vi "Actor Core.vi"(8 "error in":errorcluster, 11 "WT1600 in":refnum<class "WT1600.lvclass">) -> (0 "error out":errorcluster, 3 "Actor out":refnum<class "Actor.lvclass">)   [LabVIEW 2013, in "WT1600.lvlib" / "WT1600.lvclass"]
doc: "(<B>Filename</B>: Actor Framework.lvlib:Actor.lvclass:Actor Core.vi)\n\nReceives messages to the actor, reacts to them, and initiates any error handling that may shut the actor down.\n\nDescendant classes may override this VI to append parallel tasks for the actor to complete while it handles messages. Overrides use the Call Parent Method node."
uses:
  WT1600.lvclass
  <vilib>/ActorFramework/Actor/Actor.lvclass
  1600Card/1600Card/1600 Card Actor.lvclass
  WT1600.lvclass/WT1600.ctl
  <vilib>/ActorFramework/Actor/Actor.lvclass/Actor.ctl
  <vilib>/ActorFramework/Message Enqueuer/Message Enqueuer.lvclass/Message Enqueuer.ctl
  Observer Pattern Actor Template/Subject/Subject.lvclass
  1600Card/1600Card/1600 Card Actor.lvclass/1600 Card Actor.ctl
  Observer Pattern Actor Template/Subject Messages/Register Observer Msg/Register Observer Msg.lvclass/Register Observer Msg.ctl
  <vilib>/ActorFramework/Message Enqueuer/Init from Existing Queue.vi
  <vilib>/ActorFramework/Message Enqueuer/Enqueue.vi
  <vilib>/ActorFramework/Message Priority Queue/Priority Enqueue.vi
  <vilib>/ActorFramework/Message Enqueuer/Message Enqueuer.lvclass
  WT1600 Messages/Measure Msg/Measure Msg.lvclass
  Observer Pattern Actor Template/Subject Messages/Register Observer Msg/Register Observer Msg.lvclass
  WT1600.lvlib
panel:
  out "W-Hr":dbl
  out "Freq.":dbl
  out "Power":dbl
  out "Current":dbl
  out "Voltage":dbl
  in  "Card Number":u8=1 max=1
  in  "Array":dbl[](array[numeric])
  in  "Card Cluster":T1
  in  "New Card":bool
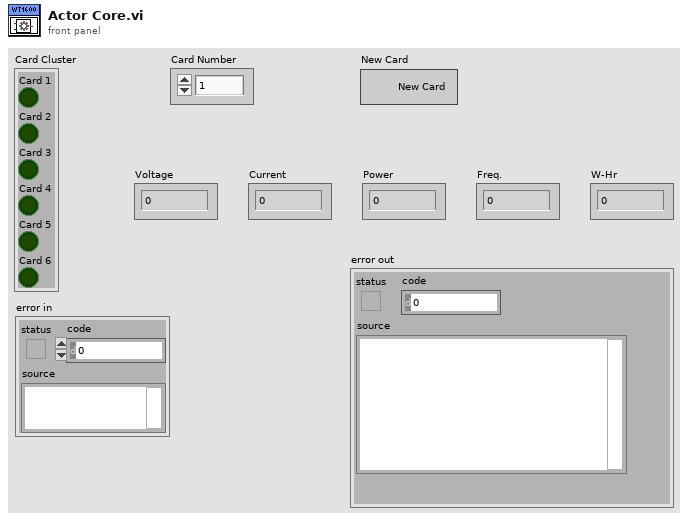
[diagram p1: front panel]
types:
  T1 = cluster{"Card 1":bool, "Card 2":bool, "Card 3":bool, "Card 4":bool, "Card 5":bool, "Card 6":bool}
  T2 = cluster{"Card Cluster[0]":bool, "Card Cluster[1]":bool, "Card Cluster[2]":bool, "Card Cluster[3]":bool, "Card Cluster[4]":bool, "Card Cluster[5]":bool}
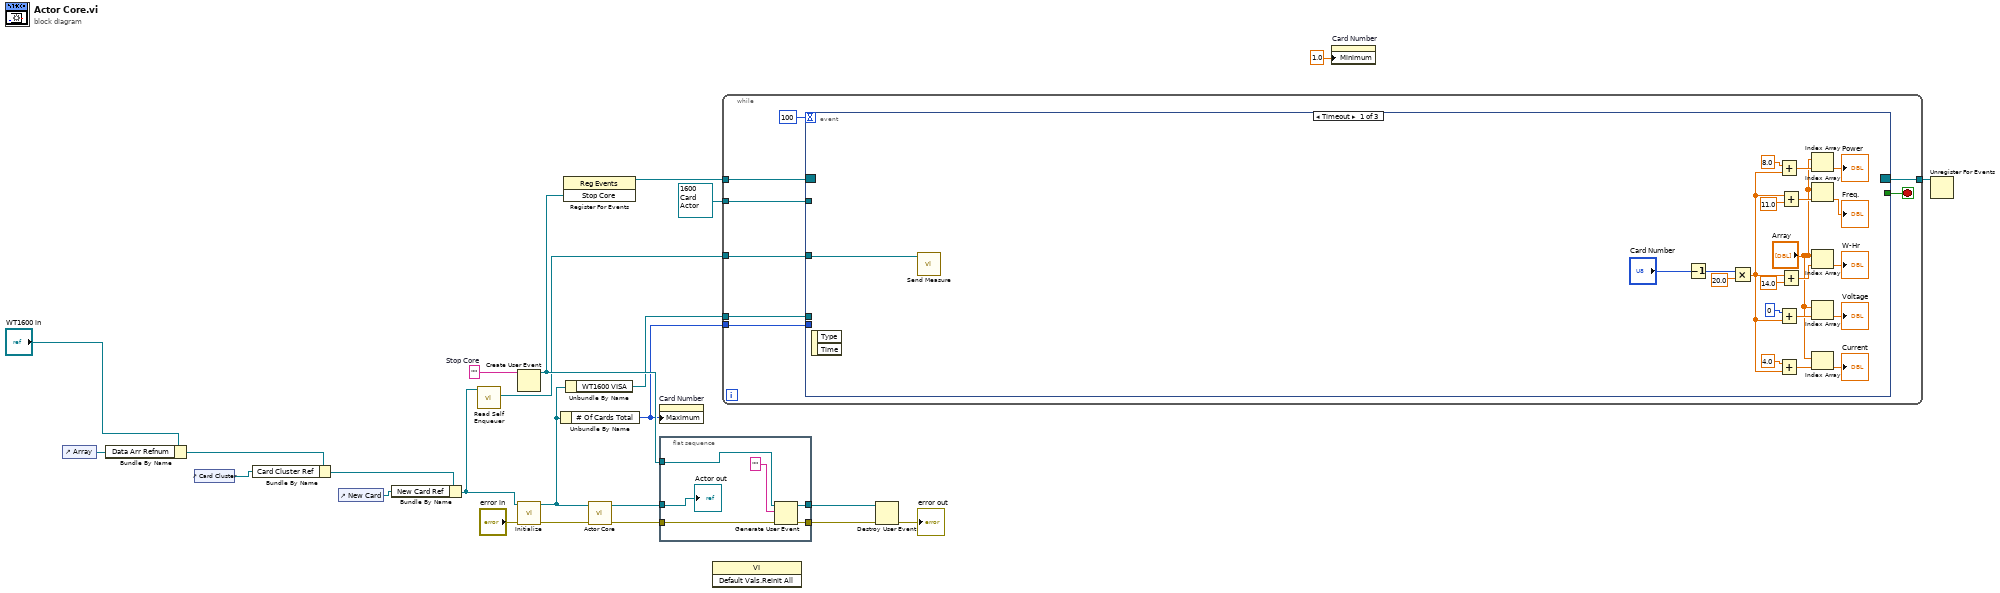
[diagram p0: block diagram]
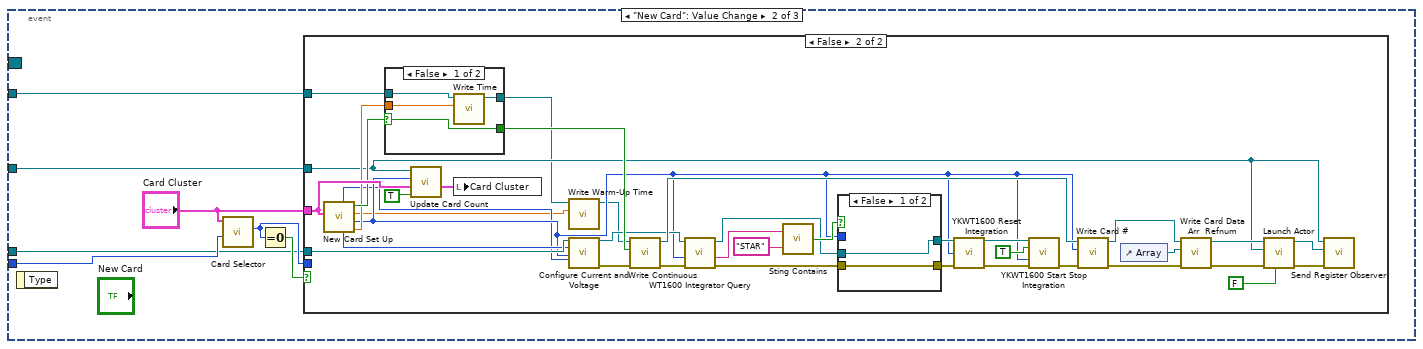
[diagram p2: hidden frame]
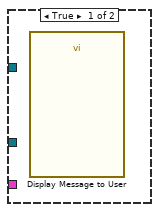
[diagram p3: hidden frame]
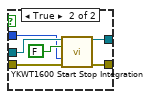
[diagram p5: hidden frame]
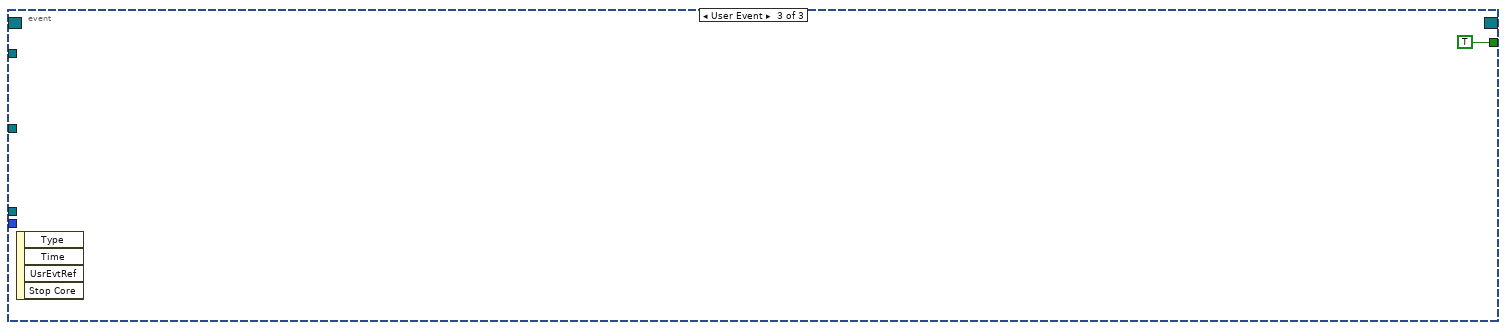
[diagram p6: hidden frame]
diagram:
  w17 = ""  # Stop Core
  n1 = control-ref of="Array"() -> (w5:refnum<vi>)
  n2 = Bundle By Name(cluster="WT1600 in", "Data Arr Refnum"=w5) -> (w6:refnum<class "WT1600.lvclass">)
  n3 = control-ref of="Card Cluster"() -> (w9:refnum<vi>)
  n4 = Bundle By Name(cluster=w6, "Card Cluster Ref"=w9) -> (w10:refnum<class "WT1600.lvclass">)
  n5 = control-ref of="New Card"() -> (w11:refnum<vi>)
  n6 = Bundle By Name(cluster=w10, "New Card Ref"=w11) -> (w8:refnum<class "WT1600.lvclass">)
  n7 = call <vilib>:"Read Self Enqueuer.vi"("Actor"=w8) -> ("Self Enqueuer"=w13:refnum<class "Message Enqueuer.lvclass">)  [unwired: 10 in]
  n8 = Create User Event(user event datatype=w17) -> (user event=w15:refnum<user-event>)  [unwired: 1 in, 1 out]
  n9 = call-dynamic "Initialize.vi"("WT1600.lvlib:WT1600.lvclass"=w8, "error in (no error)"="error in") -> ("WT1600.lvlib:WT1600.lvclass"=w3:refnum<class "WT1600.lvclass">, "error out (no error)"=w23:errorcluster)  [unwired: 11 in, 1 out]
  n10 = Unbundle By Name(w3) -> ("# Of Cards Total"=w1:i32)
  n11 = register-events(w15) -> (reference out=w16:refnum<event-registration>)  [unwired: 2 in, 1 out]
  n12 = Unbundle By Name(w3) -> ("WT1600 VISA"=w2:refnum<visa-resource-name>)
  n13 = call-parent "Actor Core.vi"("error in"=w23, "Actor in"=w3) -> ("error out"=w22:errorcluster, "Actor out"=w21:refnum<class "Actor.lvclass">)  [unwired: 8 in]
  n14 = property on="Card Number" class="DigNum (strict)"("Maximum"=w1) -> ()  [unwired: 2 in, 2 out]
  n15 = flat-sequence {
    tunnel: w22 -> [w27]
    tunnel: w21 -> [w30]
    tunnel: [w29] -> w20
    tunnel: [w28] -> w19
    tunnel: w15 -> [w26]
    frame #0 {
      n16 = Generate User Event(user event=w26, event data cluster="" ("event data"), error in=w27) -> (user event out=w29:refnum<user-event>, error out=w28:errorcluster)  [unwired: 1 in]
      "Actor out" <- w30
    }
  }
  n17 = invoke class="VI" method="Default Vals.Reinit All"() -> ()  [unwired: 3 in, 3 out]
  n18 = while {
    tunnel: w16 -> [w38]
    tunnel: [w37] -> w14
    tunnel: w13 -> [w33]
    tunnel: refnum<class "1600 Card Actor.lvclass"> refnum ("WT1600.lvlib:1600Card.lvlib:1600 Card Actor.lvclass") -> [w34]
    tunnel: w1 -> [w32]
    tunnel: w2 -> [w31]
    stop <- w36 stop-if-true
    n19 = event shown="[0] Timeout" {
      selector: w38 -> [_ _ _]
      dyn-events: [_ _ _] -> w37
      timeout: 100 -> [_ _ _]
      tunnel: [_ _ TRUE] -> w36
      tunnel: w34 -> [_ w66 _]
      tunnel: w33 -> [w59 w65 _]
      tunnel: w32 -> [_ w63 _]
      tunnel: w31 -> [_ w60 _]
      event Timeout {
        n20 = event-data() -> ()  [unwired: 1 in, 2 out]
        n21 = call "Send Measure.vi"("Message Enqueuer"=w59) -> ()  [unwired: 9 in, 2 out]
        n22 = Decrement(x="Card Number") -> (x-1=w58:u8)
        n23 = Multiply(x=w58, y=20.0) -> (x*y=w49:dbl)
        n24 = Add(x=8.0, y=w49) -> (x+y=w51:dbl)
        n25 = Add(x=0 ("index"), y=w49) -> (x+y=w54:dbl)
        n26 = Add(x=4.0, y=w49) -> (x+y=w53:dbl)
        n27 = Add(x=w49, y=11.0) -> (x+y=w47:dbl)
        n28 = Add(x=w49, y=14.0) -> (x+y=w46:dbl)
        n29 = Index Array(array="Array", index=w51) -> (element=→"Power":dbl)
        n30 = Index Array(array="Array", index=w47) -> (element=→"Freq.":dbl)
        n31 = Index Array(array="Array", index=w46) -> (element=→"W-Hr":dbl)
        n32 = Index Array(array="Array", index=w54) -> (element=→"Voltage":dbl)
        n33 = Index Array(array="Array", index=w53) -> (element=→"Current":dbl)
      }
      event "New Card": Value Change {
        n34 = event-data() -> ()  [unwired: 1 in, 1 out]
        n35 = call "Card Selector.vi"("# Of Cards Total"=w63, "Card Cluster"="Card Cluster") -> ("Card to use"=w62:i32)  [unwired: 9 in]
        n36 = Equal To 0?(x=w62) -> (x = 0?=w64:bool)
        n37 = case shown="False" w64 {
          tunnel: w66 -> [_ w77]
          tunnel: w65 -> [_ w76]
          tunnel: w62 -> [_ _]
          tunnel: "Card Cluster" -> [_ w97]
          tunnel: w60 -> [_ w75]
          frame True {
            n38 = call "Display Message to User"() -> ()  [unwired: 10 in, 2 out]
          }
          frame False {
            n39 = call "New Card Set Up.vi"("Card Cluster"=w97) -> ("Measurement Time 2"=w78:dbl, "Card chosen"=w71:i32, "Warm Up Time 2"=w67:dbl, "Continuous?"=w80:bool, "V Range (12: 1000) 2"=w72:u16, "A Range (9: 5A) 2"=w70:u16)  [unwired: 5 in]
            n40 = case shown="False" w80 {
              selector: w80 -> [w108 w110]
              tunnel: [w108 w110] -> w79
              tunnel: w78 -> [w107 _]
              tunnel: w77 -> [w106 w109]
              tunnel: [w105 w109] -> w69
              frame False {
                n41 = call "Write Time .vi"("Time"=w107, "1600 Card Actor in"=w106) -> ("1600 Card Actor out"=w105:refnum<class "1600 Card Actor.lvclass">)  [unwired: 8 in, 1 out]
              }
              frame True {
              }
            }
            n42 = call "Update Card Count.vi"("new element/subarray"=TRUE ("Open Actor Core front panel? (F)"), "cluster in"=w97, "# in"=w71, "Message Enqueuer"=w76) -> ("cluster out"=w102:T2)  [unwired: 7 in]
            n43 = local write "Card Cluster"(w102) -> ()
            n44 = call "Write Warm-Up Time.vi"("Warm-Up Time"=w67, "1600 Card Actor in"=w69) -> ("1600 Card Actor out"=w68:refnum<class "1600 Card Actor.lvclass">)  [unwired: 8 in, 1 out]
            n45 = call "Configure Current and Voltage.vi"("VISA session"=w75, "V Range (12: 1000)"=w72, "Element (0: All)"=w71, "A Range (9: 5A)"=w70) -> ("dup VISA session"=w74:refnum<visa-resource-name>, "error out"=w73:errorcluster)  [unwired: 10 in]
            n46 = call "Write Continuous"("error in (no error)"=w73, "Continuous?"=w79, "1600 Card Actor in"=w68) -> ("error out"=w81:errorcluster, "1600 Card Actor out"=w82:refnum<class "1600 Card Actor.lvclass">)  [unwired: 7 in]
            n47 = call "WT1600 Integrator Query.vi"("error in (no error)"=w81, "Element"=w71, "VISA resource name"=w74) -> ("error out"=w92:errorcluster, "Response"=w96:string, "VISA resource name out"=w93:refnum<visa-resource-name>)  [unwired: 6 in]
            n48 = call "Sting Contains.vi"("Expression to evaluate"="STAR", "Input String"=w96) -> ("Boolean"=w94:bool)
            n49 = case shown="False" w94 {
              tunnel: w93 -> [w112 w117]
              tunnel: w92 -> [w111 w116]
              tunnel: w71 -> [_ w115]
              tunnel: [w112 w114] -> w91
              tunnel: [w111 w113] -> w90
              frame False {
              }
              frame True {
                n50 = call <instrlib>:"YKWT1600 Start Stop Integration.vi"("VISA session"=w117, "Start/Stop (F: Stop)"=FALSE, "Element (All: 0)"=w115, "error in (no error)"=w116) -> ("dup VISA session"=w114:refnum<visa-resource-name>, "error out"=w113:errorcluster)  [unwired: 10 in]
              }
            }
            n51 = call <instrlib>:"YKWT1600 Reset Integration.vi"("VISA session"=w91, "Element (All: 0)"=w71, "error in (no error)"=w90) -> ("dup VISA session"=w89:refnum<visa-resource-name>, "error out"=w88:errorcluster)  [unwired: 11 in]
            n52 = call <instrlib>:"YKWT1600 Start Stop Integration.vi"("VISA session"=w89, "Start/Stop (F: Stop)"=TRUE, "Element (All: 0)"=w71, "error in (no error)"=w88) -> ("error out"=w87:errorcluster)  [unwired: 10 in, 1 out]
            n53 = call "Write Card #.vi"("error in (no error)"=w87, "Card #"=w71, "1600 Card Actor in"=w82) -> ("error out"=w85:errorcluster, "1600 Card Actor out"=w101:refnum<class "1600 Card Actor.lvclass">)  [unwired: 7 in]
            n54 = control-ref of="Array"() -> (w99:refnum<vi>)
            n55 = call "Write Card Data Arr  Refnum.vi"("error in (no error)"=w85, "Card Data Arr  Refnum"=w99, "1600 Card Actor in"=w101) -> ("error out"=w84:errorcluster, "1600 Card Actor out"=w100:refnum<class "1600 Card Actor.lvclass">)  [unwired: 7 in]
            n56 = call <vilib>:"Launch Actor.vi"("Open Actor Core front panel? (F)"=FALSE, "error in (no error)"=w84, "Actor-to-Caller Enqueuer"=w76, "Actor"=w100) -> ("error out"=w103:errorcluster, "Caller-To-Actor Enqueuer"=w104:refnum<class "Message Enqueuer.lvclass">)  [unwired: 6 in]
            n57 = call "Send Register Observer.vi"("error in (no error)"=w103, "Observer"=w104, "Message Enqueuer"=w76) -> ()  [unwired: 7 in, 2 out]
          }
        }
      }
      event User Event {
        n58 = event-data() -> ()  [unwired: 1 in, 4 out]
      }
    }
  }
  n59 = Destroy User Event(user event=w20, error in=w19) -> (error out=→"error out":errorcluster)
  n60 = property on="Card Number" class="DigNum (strict)"("Minimum"=1.0 ("Data Entry Limits:Minimum")) -> ()  [unwired: 2 in, 2 out]
  n61 = Unregister For Events(event registration refnum=w14) -> ()  [unwired: 1 in, 1 out]
